vi "CheckOverThreshold16Int.vi"(0 "Value":i16, 2 "Enable":bool, 3 "ResetAlarm":bool, 5 "Threshold":i16, 7 "TimeOut":u32) -> (4 "Alarm":bool)   [LabVIEW 2019]
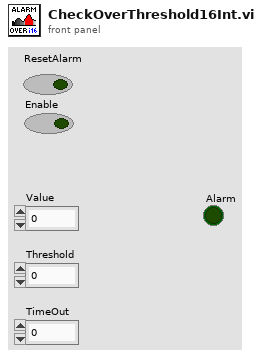
[diagram p1: front panel]
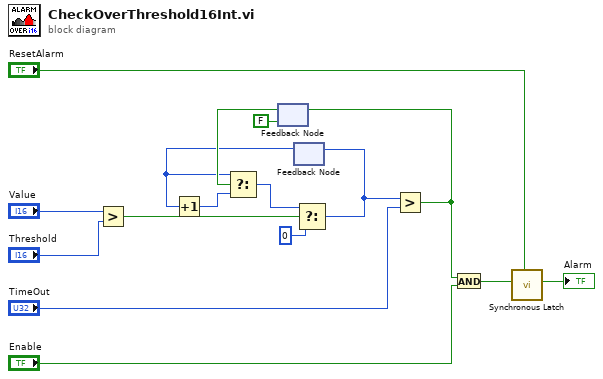
[diagram p0: block diagram]
diagram:
  n1 = Greater?(x="Value", y="Threshold") -> (0:w5:bool)
  n2 = feedback #1(FALSE) -> (w4:bool)
  n3 = feedback #2() -> (w3:u32)  [unwired: 1 in]
  n4 = Increment(x=w3) -> (x+1=w2:u32)
  n5 = Select(t=w3, s=w4, f=w2) -> (s? t:f=w1:u32)
  n6 = Select(t=w1, s=w5, f=u32 0) -> (s? t:f=w8:u32)
  n7 = feedback-in #2(w8) -> ()
  n8 = Greater?(x=w8, y="TimeOut") -> (0:w7:bool)
  n9 = feedback-in #1(w7) -> ()
  n10 = And(x=w7, y="Enable") -> (x .and. y?=w11:bool)
  n11 = call "Synchronous Latch.vi"("reset"="ResetAlarm", "set"=w11) -> ("out"=→"Alarm":bool)  [unwired: 9 in]
